vi "file -- 9data path.vi"(11 "sweep folder":path) -> (3 "9data path":path)   [LabVIEW 2014]
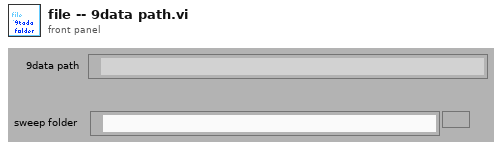
[diagram p1: front panel]
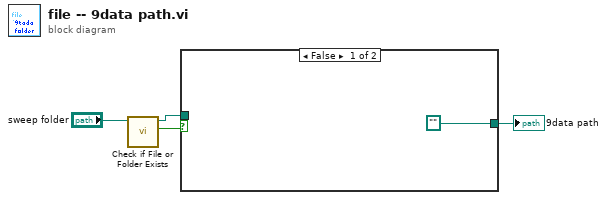
[diagram p0: block diagram]
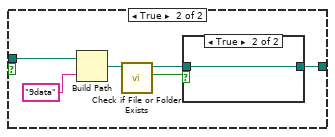
[diagram p2: hidden frame]
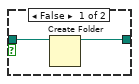
[diagram p3: hidden frame]
diagram:
  n1 = call <vilib>:"Check if File or Folder Exists.vi"("path"="sweep folder") -> ("file or folder exists?"=w3:bool, "dup path"=w2:path)  [unwired: 8 in, 1 out]
  n2 = case shown="False" w3 {
    tunnel: w2 -> [_ w10]
    tunnel: [path "" w6] -> w1
    frame False {
    }
    frame True {
      n3 = Build Path(base path=w10, name or relative path="9data" ("delimiter (\\t)")) -> (appended path=w11:path)
      n4 = call <vilib>:"Check if File or Folder Exists.vi"("path"=w11) -> ("file or folder exists?"=w8:bool, "dup path"=w7:path)  [unwired: 8 in, 1 out]
      n5 = case shown="True" w8 {
        tunnel: w7 -> [w13 w14]
        tunnel: [w12 w14] -> w6
        frame False {
          n6 = Create Folder(path (use dialog)=w13) -> (created path=w12:path)  [unwired: 2 in, 2 out]
        }
        frame True {
        }
      }
    }
  }
  "9data path" <- w1
